vi "Update Element JSON.vi"(7 "Pretty Print (T)":bool=TRUE, 8 "error in (no error)":errorcluster, 9 "JSON":string, 11 "Ctl Refnum in":refnum<vi>) -> (0 "error out":errorcluster, 3 "Ctl Refnum":refnum<vi>)   [LabVIEW 2020, in "VolatusGUIControls.lvlib"]
uses:
  VolatusGUIControls.lvlib
  <vilib>/JDP Science/JSONtext/JSONtext.lvlib
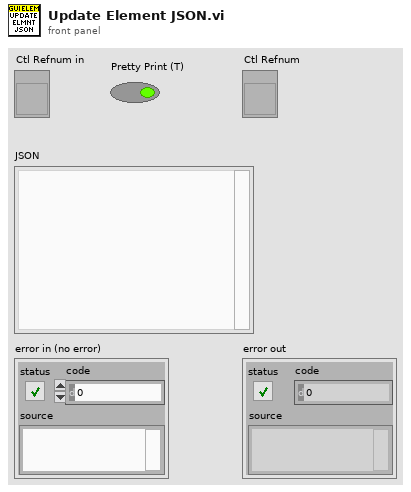
[diagram p1: front panel]
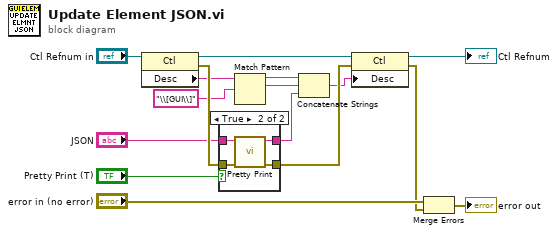
[diagram p0: block diagram]
diagram:
  n1 = property class="Ctl"(reference="Ctl Refnum in") -> (reference out=w7:refnum<vi>, error out=w15:errorcluster, "Desc"=w14:string)  [unwired: 1 in]
  n2 = case shown="True" "Pretty Print (T)" {
    tunnel: [w17 w22] -> w16
    tunnel: w15 -> [w17 w21]
    tunnel: "JSON" -> [w18 w20]
    tunnel: [w18 w19] -> w8
    frame False {
    }
    frame True {
      n3 = call <vilib>:"Pretty Print.vi"("error in (no error)"=w21, "JSON"=w20) -> ("error out"=w22:errorcluster, "<JSON>"=w19:string)  [unwired: 7 in, 1 out]
    }
  }
  n4 = Match Pattern(string=w14, regular expression="\\[GUI\\]") -> (before substring=w11:string, match substring=w10:string)  [unwired: 1 in, 2 out]
  n5 = Concatenate Strings(w11, w10, w8) -> (w6:string)
  n6 = property class="Ctl"(reference=w7, error in=w16, "Desc"=w6) -> (reference out=→"Ctl Refnum":refnum<vi>, error out=w3:errorcluster)
  n7 = Merge Errors("error in (no error)", w3) -> (→"error out":errorcluster)
